vi "Read Configuration Data.vi"(0 "Lock-In Variable Channels in":refnum<class "Lock-In Variable Channels_2.lvclass">, 7 "error in (no error)":errorcluster) -> (16 "Max AI Rate":i32, 17 "Auto Control Max AI Rate/AI Block Size":bool, 19 "Input Signals":i16, 20 "Lock-In Variable Channels out":refnum<class "Lock-In Variable Channels_2.lvclass">, 21 "AO Configuration":T3(array[cluster]), 22 "OSC Configuration":T2(array[cluster]), 23 "AI Configuration":T4(array[cluster])=[{"AI.Coupling"=10050, "AI.Max"=10.0, "AI.Min"=-10.0, "Input physical channels"="PXI1Slot2/ai0:1"}, {"AI.Coupling"=10050, "AI.Max"=10.0, "AI.Min"=-10.0, "Input physical channels"="PXI1Slot3/ai0:1"}, {"AI.Coupling"=10050, "AI.Max"=10.0, "AI.Min"=-10.0, "Input physical channels"="PXI1Slot6/ai0:1"}] {"AI.Coupling" items=["AC"=10045, "DC"=10050, "GND"=10066]}, 24 "AI Block Size":i32, 25 "AI Buffer Size (s)":i32, 26 "Phase&Tc":T1(array[cluster]), 27 "error out":errorcluster)   [LabVIEW 2013, in "Lock-In Variable Channels_2.lvclass"]
uses:
  Lock-In Variable Channels_2.lvclass
  Lock-In Variable Channels_2.lvclass/Lock-In Variable Channels_2.ctl
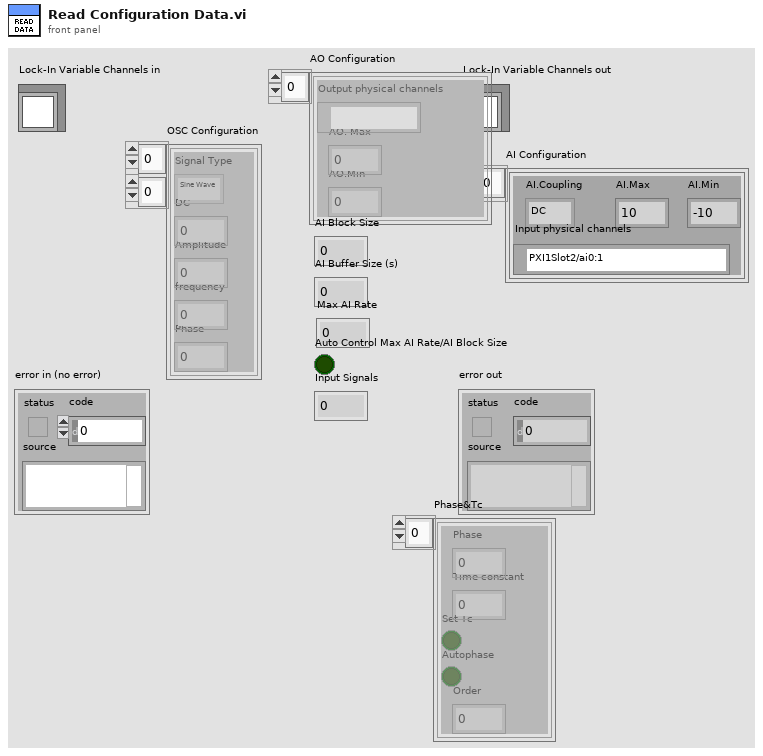
[diagram p1: front panel]
types:
  T1 = cluster{"Phase":dbl, "Time constant":dbl, "Set Tc":bool, "Autophase":bool, "Order":dbl}[]
  T2 = cluster{"Signal Type":enum16{"Sine Wave", "Triangle Wave", "Square Wave", "Sawtooth Wave"}, "DC":dbl, "Amplitude":dbl, "frequency":dbl, "Phase":dbl}[][]
  T3 = cluster{"Output physical channels":tag, "AO. Max":dbl, "AO.Min":dbl}[]
  T4 = cluster{"AI.Coupling":i32, "AI.Max":dbl, "AI.Min":dbl, "Input physical channels":tag}[]
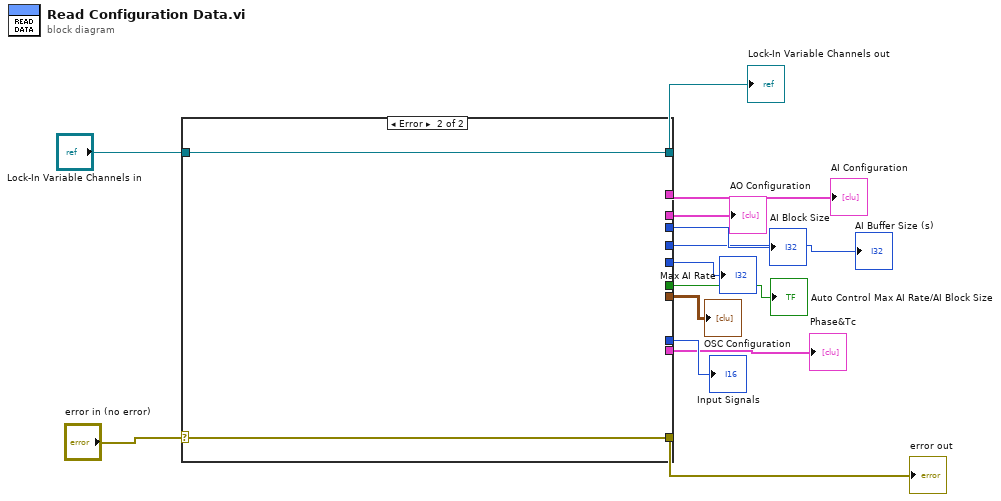
[diagram p0: block diagram]
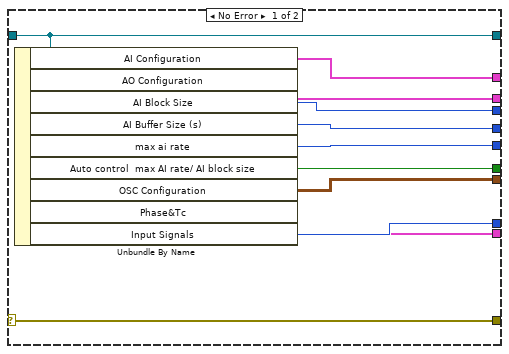
[diagram p2: hidden frame]
diagram:
  n1 = case shown="Error" "error in (no error)" {
    selector: "error in (no error)" -> [w24 w25]
    tunnel: [w24 w25] -> w12
    tunnel: [w23 w26] -> w10
    tunnel: "Lock-In Variable Channels in" -> [w23 w26]
    tunnel: [w22 _] -> w9
    tunnel: [w21 _] -> w8
    tunnel: [w20 _] -> w7
    tunnel: [w19 _] -> w6
    tunnel: [w18 _] -> w5
    tunnel: [w17 _] -> w4
    tunnel: [w16 _] -> w3
    tunnel: [w15 _] -> w2
    tunnel: [w14 _] -> w1
    frame No Error {
      n2 = Unbundle By Name(w23) -> ("AI Configuration"=w22:T4, "AO Configuration"=w21:T3, "AI Block Size"=w20:i32, "AI Buffer Size (s)"=w19:i32, "max ai rate"=w18:i32, "Auto control  max AI rate/ AI block size"=w17:bool, "OSC Configuration"=w15:T2, "Phase&Tc"=w14:T1, "Input Signals"=w16:i16)
    }
    frame Error {
    }
  }
  "error out" <- w12
  "Lock-In Variable Channels out" <- w10
  "AI Configuration" <- w9
  "AO Configuration" <- w8
  "AI Block Size" <- w7
  "AI Buffer Size (s)" <- w6
  "Max AI Rate" <- w5
  "Auto Control Max AI Rate/AI Block Size" <- w4
  "Input Signals" <- w3
  "OSC Configuration" <- w2
  "Phase&Tc" <- w1
